vi "Check Expiration.vi"(0 "Path in":refnum<class "Path.lvclass">, 11 "error in (no error)":errorcluster) -> (4 "Path out":refnum<class "Path.lvclass">, 6 "Expired?":bool, 15 "error out":errorcluster)   [LabVIEW 2023, in "RFCalAndFixtureCharact.Common.lvlib" / "Path.lvclass"]
uses:
  Path.lvclass
  Result Accessor/Result Accessor.lvclass
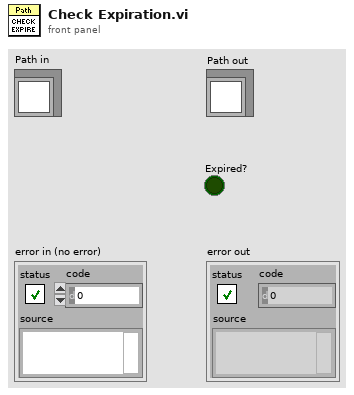
[diagram p1: front panel]
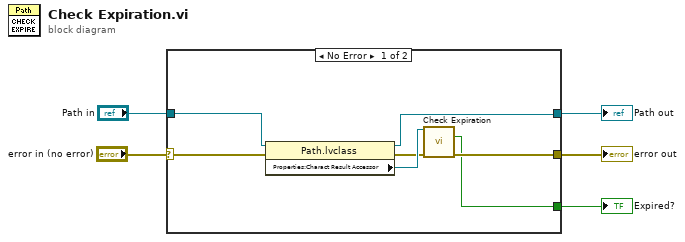
[diagram p0: block diagram]
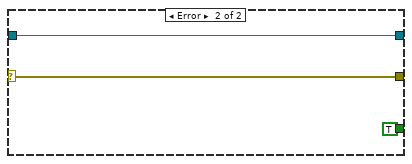
[diagram p2: hidden frame]
diagram:
  n1 = case shown="No Error" "error in (no error)" {
    selector: "error in (no error)" -> [w11 w14]
    tunnel: [w6 TRUE] -> w5
    tunnel: [w8 w14] -> w3
    tunnel: "Path in" -> [w12 w15]
    tunnel: [w7 w15] -> w1
    frame No Error {
      n2 = property class="Path.lvclass"(reference=w12, error in=w11) -> (reference out=w7:refnum<class "Path.lvclass">, error out=w9:errorcluster, "Properties:Charact Result Accessor"=w10:refnum<class "Result Accessor.lvclass">)
      n3 = call-dynamic "Check Expiration.vi"("Charact Result Accessor in"=w10, "error in"=w9) -> ("Expired?"=w6:bool, "error out"=w8:errorcluster)  [unwired: 11 in, 1 out]
    }
    frame Error {
    }
  }
  "Expired?" <- w5
  "error out" <- w3
  "Path out" <- w1
